vi "Thread@SubThreadWait__Parameter.vi"(1 "ParamterIn":string) -> (0 "ParamterOut":string)   [LabVIEW 2020]
panel:
  out "SubThread Name":string[](array[string])
  in  "Mode":string(combo)
  in  "Thread Label":string(combo)
  in  "Confirm":bool
  # "Thread@SubThreadWait $SubName1(,$SubName2.....)\nThread@SubThreadWait $SubName1(,$SubName2.....),SkipNotFind=1"
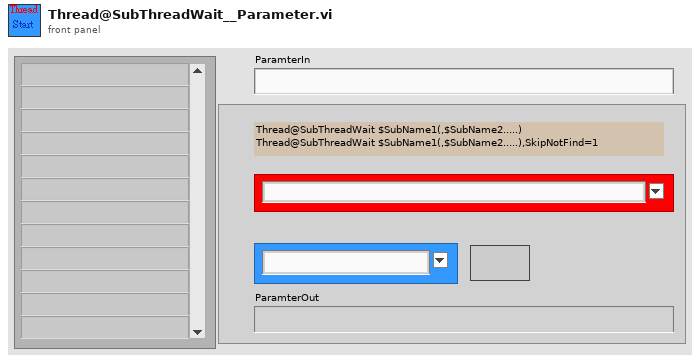
[diagram p1: front panel]
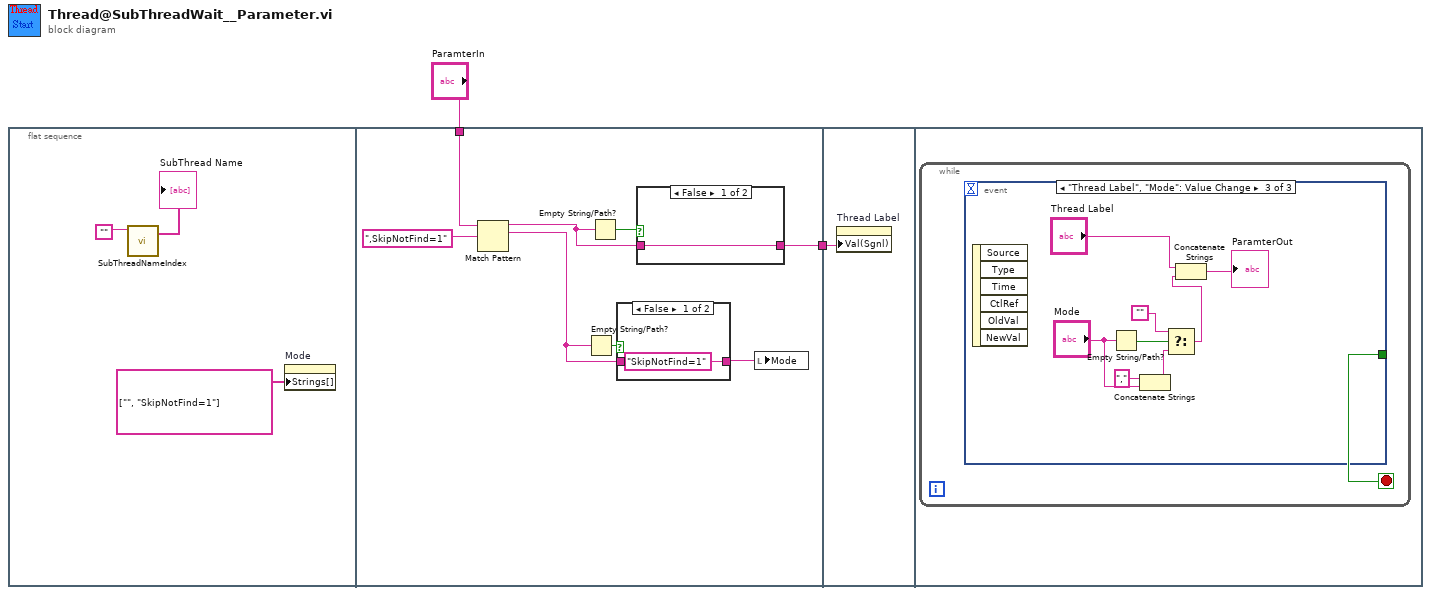
[diagram p0: block diagram]
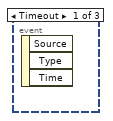
[diagram p4: hidden frame]
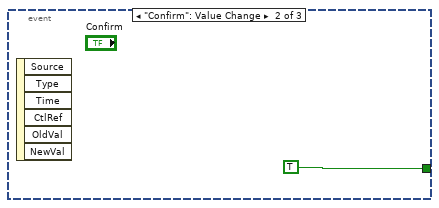
[diagram p5: hidden frame]
diagram:
  n1 = flat-sequence {
    tunnel: "ParamterIn" -> [w9]
    tunnel: [w12] -> w1
    tunnel: w1 -> [w16]
    frame #0 {
      n2 = call "SubThreadNameIndex.vi"("SubThreadName"="") -> ("SubThread Name"=→"SubThread Name":string[])  [unwired: 7 in, 3 out]
      n3 = property on="Mode" class="CmbBox"("Strings[]"=string[] ["", "SkipNotFind=1"] ("Strings []")) -> ()  [unwired: 2 in, 2 out]
    }
    frame #1 {
      n4 = Match Pattern(string=w9, regular expression=",SkipNotFind=1") -> (before substring=w7:string, match substring=w6:string)  [unwired: 1 in, 2 out]
      n5 = Empty String/Path?(string/path=w6) -> (empty?=w11:bool)
      n6 = Empty String/Path?(string/path=w7) -> (empty?=w13:bool)
      n7 = case shown="False" w11 {
        tunnel: w6 -> [_ _]
        tunnel: ["SkipNotFind=1" ("ParamterIn") _] -> w10
        frame False {
        }
        frame True {
        }
      }
      n8 = case shown="False" w13 {
        tunnel: w7 -> [w15 _]
        tunnel: [w15 _] -> w12
        frame False {
        }
        frame True {
        }
      }
      n9 = local write "Mode"(w10) -> ()
    }
    frame #2 {
      n10 = property on="Thread Label" class="CmbBox"("Val(Sgnl)"=w16) -> ()  [unwired: 2 in, 2 out]
    }
    frame #3 {
      n11 = while {
        stop <- w17 stop-if-true
        n12 = event shown="[2] \"Thread Label\", \"Mode\": Value Change" {
          selector: _ -> [_ _ _]
          dyn-events: _ -> [_ _ _]
          timeout: _ -> [_ _ _]
          tunnel: [_ TRUE _] -> w17
          event Timeout {
            n13 = event-data() -> ()  [unwired: 1 in, 3 out]
          }
          event "Confirm": Value Change {
            n14 = event-data() -> ()  [unwired: 1 in, 6 out]
          }
          event "Thread Label", "Mode": Value Change {
            n15 = event-data() -> ()  [unwired: 1 in, 6 out]
            n16 = Empty String/Path?(string/path="Mode") -> (empty?=w26:bool)
            n17 = Concatenate Strings("," ("string"), "Mode") -> (w24:string)
            n18 = Select(t="", s=w26, f=w24) -> (s? t:f=w19:string)
            n19 = Concatenate Strings("Thread Label", w19) -> (→"ParamterOut":string)
          }
        }
      }
    }
  }
